vi "Hide core.vi"(8 "error in (no error)":errorcluster, 11 "Subpanel in":refnum<class "Subpanel.lvclass">) -> (0 "error out":errorcluster)   [LabVIEW 2020, in "Panel.lvlib" / "Subpanel.lvclass"]
doc: "Removes the Panel from the subpanel.\n\n----\nPlease see the following web address for additional documentation and tutorial information:\nhttp://www.mooregoodideas.com/mgi-panel-manager/\n\nAuthor: Derek Trepanier\n\nCopyright (c) 2018, Moore Good Ideas, Inc.\n\nAll rights reserved.\n\nRedistribution and use in source and binary forms, with or without modification, are permitted provided that the following conditions are met:\n\n * Redistributions of source code must retain the above copyright notice, this list of conditions and the following disclaimer.\n * Redistributions in binary form must reproduce the above copyright notice, this list of conditions and the following disclaimer in the documentation and/or other materials provided with the distribution.\n * Neither the name of Moore Good Ideas, Inc. nor the names of its contributors may be used to endorse or promote products derived from this software without specific prior written permission.\n\nTHIS SOFTWARE IS PROVIDED BY THE COPYRIGHT HOLDERS AND CONTRIBUTORS \"AS IS\" AND ANY EXPRESS OR IMPLIED WARRANTIES, INCLUDING, BUT NOT LIMITED TO, THE IMPLIED WARRANTIES OF MERCHANTABILITY AND FITNESS FOR A PARTICULAR PURPOSE ARE DISCLAIMED. IN NO EVENT SHALL THE COPYRIGHT OWNER OR CONTRIBUTORS BE LIABLE FOR ANY DIRECT, INDIRECT, INCIDENTAL, SPECIAL, EXEMPLARY, OR CONSEQUENTIAL DAMAGES (INCLUDING, BUT NOT LIMITED TO, PROCUREMENT OF SUBSTITUTE GOODS OR SERVICES; LOSS OF USE, DATA, OR PROFITS; OR BUSINESS INTERRUPTION) HOWEVER CAUSED AND ON ANY THEORY OF LIABILITY, WHETHER IN CONTRACT, STRICT LIABILITY, OR TORT (INCLUDING NEGLIGENCE OR OTHERWISE) ARISING IN ANY WAY OUT OF THE USE OF THIS SOFTWARE, EVEN IF ADVISED OF THE POSSIBILITY OF SUCH DAMAGE."
uses:
  <vilib>/MGI/Panel Manager/Panel/Panel/Subpanel/Subpanel.lvclass
  <vilib>/MGI/Panel Manager/Panel/Panel/Subpanel/Action.ctl
  <vilib>/MGI/Panel Manager/Panel/Panel/Subpanel/Subpanel.lvclass/Subpanel.ctl
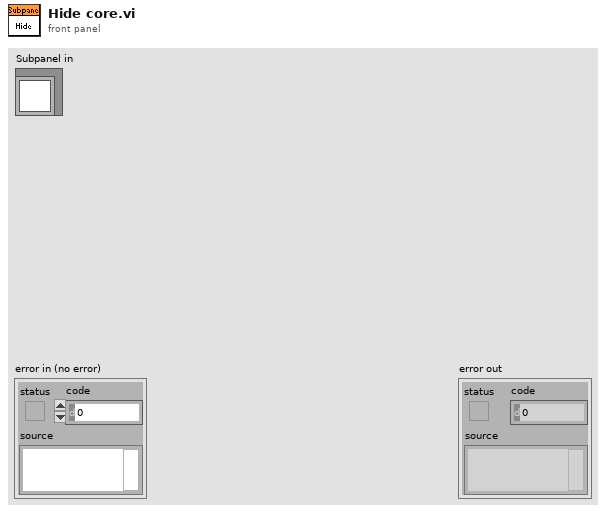
[diagram p1: front panel]
types:
  T1 = typedef "Panel.lvlib/Subpanel.lvclass/Action.ctl" = enum16{"Query", "Take", "Release"}
  T2 = typedef "Semaphore RefNum" = refnum<k1>
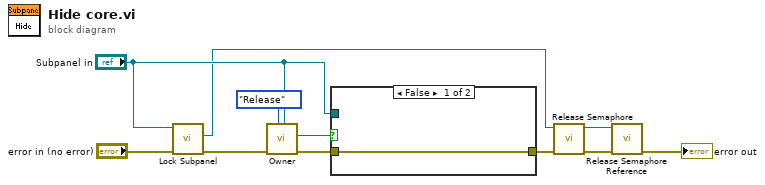
[diagram p0: block diagram]
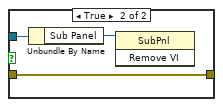
[diagram p2: hidden frame]
diagram:
  n1 = call <vilib>:"Lock Subpanel.vi"("error in (no error)"="error in (no error)", "Subpanel in"="Subpanel in") -> ("error out"=w10:errorcluster, "semaphore"=w9:T2)  [unwired: 8 in]
  n2 = call <vilib>:"Owner.vi"("Action"=Action."Release", "error in (no error)"=w10, "Subpanel in"="Subpanel in") -> ("error out"=w7:errorcluster, "I Was Owner?"=w6:bool)  [unwired: 6 in, 1 out]
  n3 = case shown="False" w6 {
    tunnel: w7 -> [w12 w15]
    tunnel: [w12 w15] -> w4
    tunnel: "Subpanel in" -> [_ w13]
    frame False {
    }
    frame True {
      n4 = Unbundle By Name(w13) -> ("Sub Panel"=w14:refnum<vi>)
      n5 = invoke class="SubPnl" method="Remove VI"(reference=w14) -> ()  [unwired: 2 in, 3 out]
    }
  }
  n6 = call <vilib>:"Release Semaphore.vi"("error in (no error)"=w4, "semaphore"=w9) -> ("error out"=w2:errorcluster, "semaphore out"=w3:T2)  [unwired: 4 in]
  n7 = call <vilib>:"Release Semaphore Reference.vi"("error in (no error)"=w2, "semaphore"=w3) -> ("error out"=→"error out":errorcluster)  [unwired: 8 in, 1 out]
